vi "Next.vi"(8 "error in (no error)":errorcluster, 10 "Query in":refnum<class "Query Result.lvclass">, 11 "SqlMapper in":refnum<class "SqlMapper.lvclass">) -> (0 "error out":errorcluster, 1 "found?":bool=TRUE, 2 "Row":variant, 3 "SqlMapper out":refnum<class "SqlMapper.lvclass">)   [LabVIEW 2020, in "ORM.lvlib" / "Query Result.lvclass"]
uses:
  Query Result.lvclass
  SqlMapper/SqlMapper.lvclass
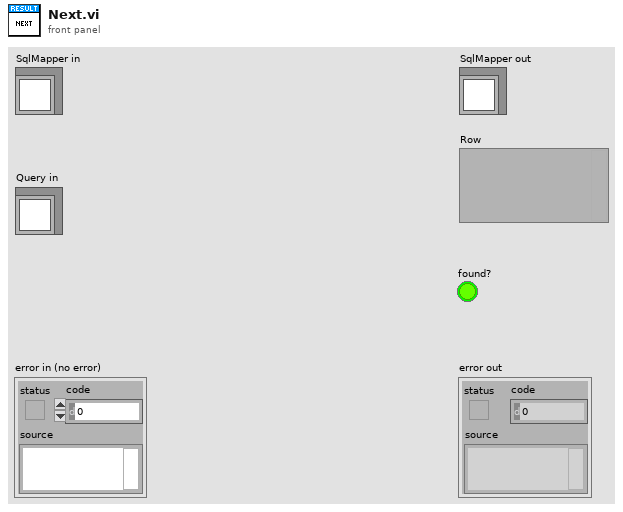
[diagram p1: front panel]
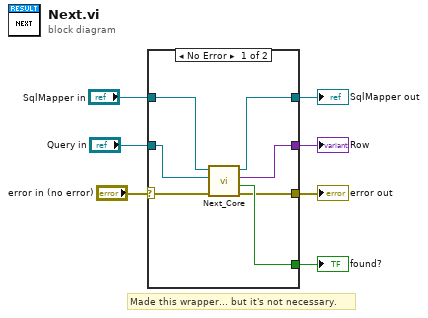
[diagram p0: block diagram]
diagram:
  # "Made this wrapper... but it's not necessary."
  n1 = case shown="No Error" "error in (no error)" {
    selector: "error in (no error)" -> [w14 w16]
    tunnel: [w8 w16] -> w6
    tunnel: "Query in" -> [w11 _]
    tunnel: [w13 _] -> w4
    tunnel: [w10 w15] -> w3
    tunnel: "SqlMapper in" -> [w12 w15]
    tunnel: [w9 _] -> w1
    frame No Error {
      n2 = call-dynamic "Next_Core.vi"("error in (no error)"=w14, "Query Result in"=w11, "SqlMapper in"=w12) -> ("error out"=w8:errorcluster, "Found"=w13:bool, "Row as Variant"=w9:variant, "SqlMapper out"=w10:refnum<class "SqlMapper.lvclass">)  [unwired: 5 in]
    }
    frame Error {
    }
  }
  "error out" <- w6
  "found?" <- w4
  "Row" <- w1
  "SqlMapper out" <- w3
